vi "Excel_Update_Chart.vi"(0 "Excel._Worksheet":refnum<k7>, 1 "chart data":dbl[][](array[numeric]) format="%0.2f", 5 "Shapes":refnum<k7>, 9 "Chart index":u16, 11 "error in (no error)":errorcluster, 12 "column header":string[](array[string]), 13 "row header":string[](array[string])) -> (15 "error out":errorcluster)   [LabVIEW 2010, in "NI_ReportGenerationToolkit.lvlib"]
uses:
  <vilib>/addons/_office/NI_ReportGenerationToolkit.lvlib
panel:
  in  "MS Graph":refnum<k7>
  in  "Excel._OLEObject":refnum<k7>
  in  "Graph.Chart":refnum<k7>
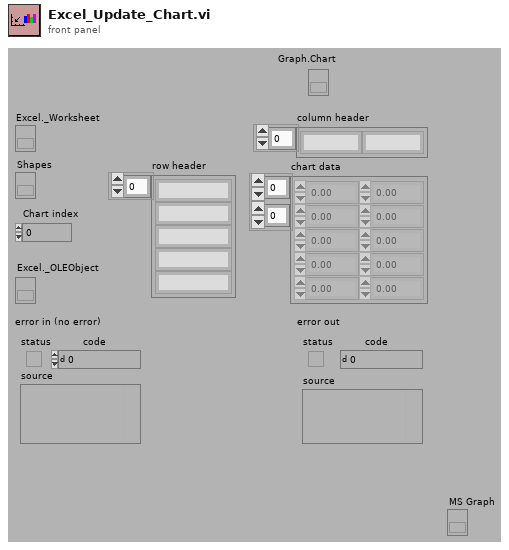
[diagram p1: front panel]
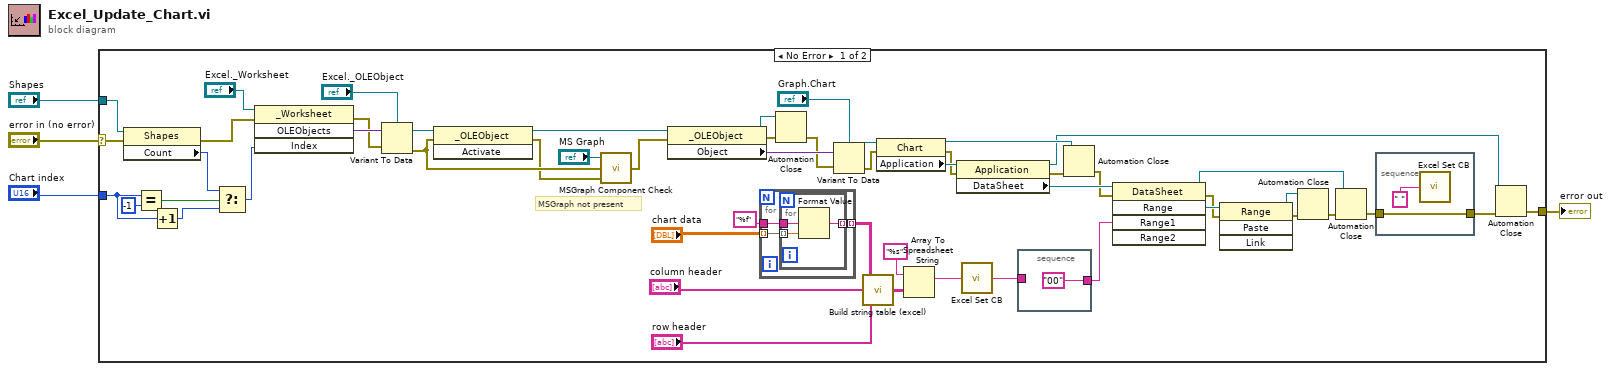
[diagram p0: block diagram]
diagram:
  n1 = case shown="No Error" "error in (no error)" {
    selector: "error in (no error)" -> [w5 w66]
    tunnel: "Chart index" -> [w44 _]
    tunnel: [w17 w66] -> w3
    tunnel: "Shapes" -> [w13 _]
    frame No Error {
      # "MSGraph not present"
      n2 = property class="Shapes"(reference=w13, error in=w5) -> (error out=w47:errorcluster, "Count"=w46:i32)  [unwired: 1 out]
      n3 = Equal?(x=w44, y=i16 -1) -> (x = y?=w55:bool)
      n4 = Increment(x=w44) -> (x+1=w53:u16)
      n5 = Select(t=w46, s=w55, f=w53) -> (s? t:f=w45:i32)
      n6 = invoke class="_Worksheet" method="OLEObjects"(reference="Excel._Worksheet", error in=w47, "Index"=w45) -> (error out=w50:errorcluster, "OLEObjects"=w51:variant)  [unwired: 1 in, 2 out]
      n7 = Variant To Data(error in=w50, Variant=w51, type="Excel._OLEObject") -> (error out=w8:errorcluster, data=w23:refnum<k7>)
      n8 = invoke class="_OLEObject" method="Activate"(reference=w23, error in=w8) -> (reference out=w22:refnum<k7>, error out=w7:errorcluster)  [unwired: 1 in, 1 out]
      n9 = call <vilib>:"MSGraph Component Check.vi"("error 2"=w7, "error 1"=w8, "MS Graph"="MS Graph") -> ("error out"=w6:errorcluster)
      n10 = property class="_OLEObject"(reference=w22, error in=w6) -> (reference out=w48:refnum<k7>, error out=w49:errorcluster, "Object"=w43:variant)
      n11 = for {
        tunnel: "chart data" -> [w62] mode=indexing
        tunnel: "%f" -> [w61]
        tunnel: [w60] -> w40 mode=indexing
        n12 = for {
          tunnel: w62 -> [w65] mode=indexing
          tunnel: w61 -> [w64]
          tunnel: [w63] -> w60 mode=indexing
          n13 = Format Value(format string=w64, value (0)=w65) -> (output string=w63:string)  [unwired: 1 out]
        }
      }
      n14 = Automation Close(3:w49, 5:w48) -> (0:w42:errorcluster)
      n15 = Variant To Data(error in=w42, Variant=w43, type="Graph.Chart") -> (error out=w41:errorcluster, data=w12:refnum<k7>)
      n16 = call <vilib>:"Build string table (excel).vi"("row headers"="row header", "column headers"="column header", "text data"=w40) -> ("output table"=w38:string[][])
      n17 = property class="Chart"(reference=w12, error in=w41) -> (reference out=w26:refnum<k7>, error out=w25:errorcluster, "Application"=w27:refnum<k7>)
      n18 = Array To Spreadsheet String(array=w38, 3:"%s" ("format string")) -> (spreadsheet string=w11:string)  [unwired: 1 out]
      n19 = property class="Application"(reference=w27, error in=w25) -> (reference out=w15:refnum<k7>, error out=w18:errorcluster, "DataSheet"=w30:refnum<k7>)
      n20 = call <vilib>:"Excel Set CB.vi"("String"=w11) -> ("String 2"=w10:string)
      n21 = stacked-sequence {
        tunnel: ["00"] -> w20
        tunnel: w10 -> [_]
        frame #0 {
        }
      }
      n22 = Automation Close(3:w18, 5:w26) -> (0:w29:errorcluster)
      n23 = invoke class="DataSheet" method="Range"(reference=w30, error in=w29, "Range1"=w20) -> (reference out=w32:refnum<k7>, error out=w31:errorcluster, "Range"=w33:refnum<k7>)  [unwired: 2 in, 2 out]
      n24 = invoke class="Range" method="Paste"(reference=w33, error in=w31) -> (reference out=w35:refnum<k7>, error out=w36:errorcluster)  [unwired: 2 in, 2 out]
      n25 = Automation Close(3:w36, 5:w35) -> (0:w34:errorcluster)
      n26 = Automation Close(3:w34, 5:w32) -> (0:w28:errorcluster)
      n27 = stacked-sequence {
        tunnel: w28 -> [w59]
        tunnel: [w59] -> w16
        frame #0 {
          n28 = call <vilib>:"Excel Set CB.vi"("String"=" ") -> ()  [unwired: 1 out]
        }
      }
      n29 = Automation Close(3:w16, 5:w15) -> (0:w17:errorcluster)
    }
    frame Error {
    }
  }
  "error out" <- w3
